vi "CH_LM App DisplayDataFromFile.vi"(0 "Path":path) -> ()   [LabVIEW 2012, in "CH_LM App.lvlib"]
doc: "This VI opens a data file reads the contents and displays them on the frontpanel."
uses:
  CH_LM App.lvlib
  <vilib>/Analysis/NI_AALBase.lvlib
  CH_LM.lvlib
panel:
  out "Table":string[][](table)
  out "Statistics":T1 {"Max" format="%#_4p"; "Min" format="%#_4p"; "Std.Dev." format="%#_4p"; "Mean" format="%#_4p"}
  in  "column":u8
  in  "Statistics Type":T2 {"Max" format="%#_4p"; "Min" format="%#_4p"; "Std. Dev." format="%#_4p"; "Mean" format="%#_4p"}
  out "Statistics Array":T3(array[cluster]) {"Max" format="%#_4p"; "Min" format="%#_4p"; "Std. Dev." format="%#_4p"; "Mean" format="%#_4p"}
  out "Waveform Graph":dbl[][](graph)
  in  "Print":bool
  out "Date and Time":string
  in  "Close":bool
  out "Data file":path
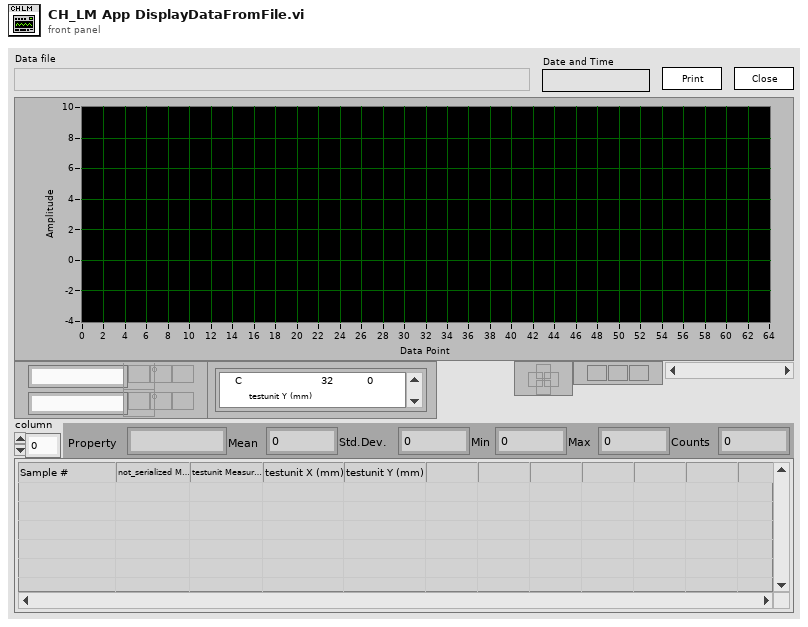
[diagram p1: front panel]
types:
  T1 = cluster{"Property":string, "Mean":dbl, "Std.Dev.":dbl, "Min":dbl, "Max":dbl, "Counts":i32}
  T2 = cluster{"Serial":string, "Mean":dbl, "Std. Dev.":dbl, "Min":dbl, "Max":dbl, "Counts":i32}
  T3 = cluster{"Serial":string, "Mean":dbl, "Std. Dev.":dbl, "Min":dbl, "Max":dbl, "Counts":i32}[]
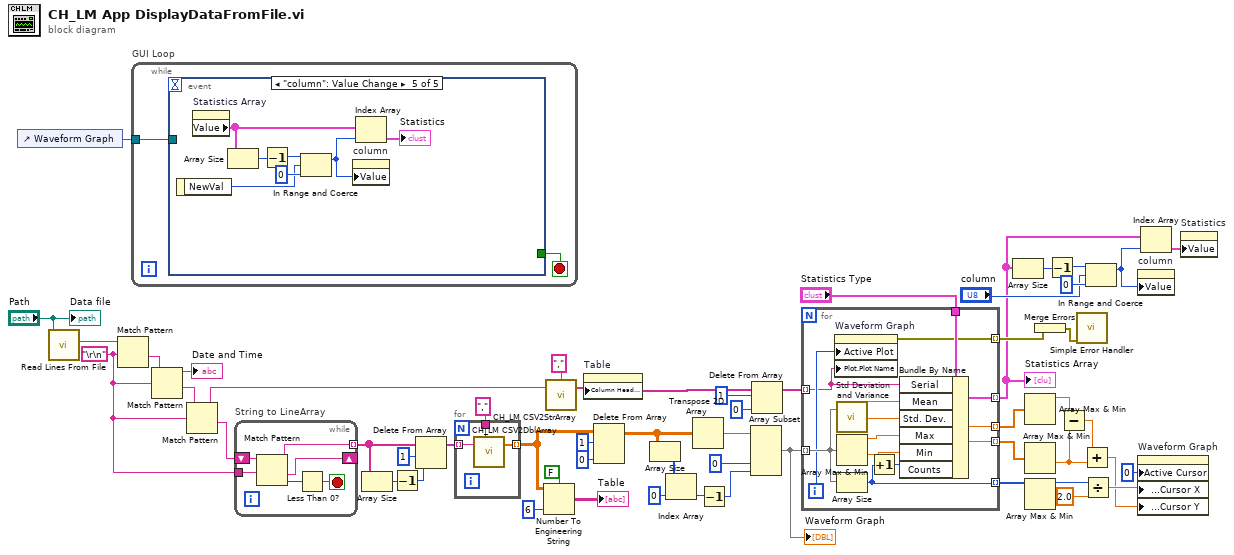
[diagram p0: block diagram]
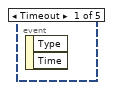
[diagram p2: hidden frame]
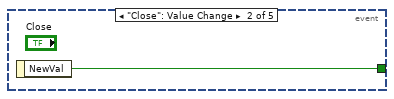
[diagram p3: hidden frame]
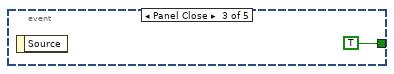
[diagram p4: hidden frame]
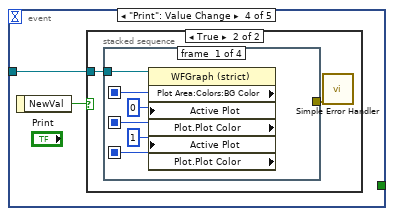
[diagram p5: hidden frame]
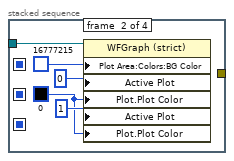
[diagram p7: hidden frame]
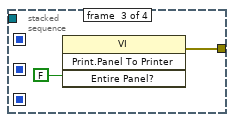
[diagram p8: hidden frame]
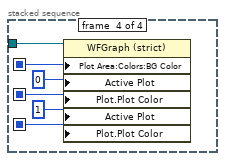
[diagram p9: hidden frame]
diagram:
  w19 = "\r\n" ("End of Line Constant")
  n1 = control-ref of="Waveform Graph"() -> (w50:refnum<vi>)
  n2 = call <vilib>:"Read Lines From File.vi"("file path (dialog if empty)"="Path") -> ("line string"=w54:string)  [unwired: 1 in, 7 out]
  n3 = Match Pattern(string=w54, regular expression=w19) -> (after substring=w53:string)  [unwired: 4 out]
  n4 = while "GUI Loop" {
    tunnel: w50 -> [w56]
    stop <- w57 stop-if-true
    n5 = event shown="[4] \"column\": Value Change" {
      selector: _ -> [_ _ _ _ _]
      dyn-events: _ -> [_ _ _ _ _]
      timeout: _ -> [_ _ _ _ _]
      tunnel: [_ w58 TRUE ("NewVal") _ _] -> w57
      tunnel: w56 -> [_ _ _ w60 _]
      event Timeout {
        n6 = event-data() -> ()  [unwired: 3 out]
      }
      event "Close": Value Change {
        n7 = event-data() -> ("NewVal"=w58:bool)  [unwired: 1 out]
      }
      event Panel Close {
        n8 = event-data() -> ()  [unwired: 2 out]
      }
      event "Print": Value Change {
        n9 = event-data() -> ("NewVal"=w61:bool)  [unwired: 1 out]
        n10 = case shown="True" w61 {
          tunnel: w60 -> [_ w62]
          frame False {
          }
          frame True {
            n11 = stacked-sequence {
              seq-local: [w66 _ _ _] -> [_ _ _ w81]
              seq-local: [w65 _ _ _] -> [_ _ _ w79]
              seq-local: [w64 _ _ _] -> [_ _ _ w77]
              tunnel: [_ _ w75 _] -> w63
              tunnel: w62 -> [w69 w74 _ w82]
              frame #0 {
                n12 = property class="WFGraph (strict)"(reference=w69, "Active Plot"=u32 0, "Active Plot"=u32 1) -> ("Plot Area:Colors:BG Color"=w66:u32, "Plot.Plot Color"=w65:u32, "Plot.Plot Color"=w64:u32)  [unwired: 1 in, 2 out]
              }
              frame #1 {
                w70 = u32 0 ("Plot Area:Colors:BG Color")
                n13 = property class="WFGraph (strict)"(reference=w74, "Plot Area:Colors:BG Color"=u32 16777215, "Active Plot"=u32 0, "Plot.Plot Color"=w70, "Active Plot"=u32 1, "Plot.Plot Color"=w70) -> ()  [unwired: 1 in, 2 out]
              }
              frame #2 {
                n14 = invoke on="Invoke Node" class="VI" method="Print.Panel To Printer"("Entire Panel?"=FALSE) -> (error out=w75:errorcluster)  [unwired: 3 in, 3 out]
              }
              frame #3 {
                n15 = property class="WFGraph (strict)"(reference=w82, "Plot Area:Colors:BG Color"=w81, "Active Plot"=u32 0, "Plot.Plot Color"=w79, "Active Plot"=u32 1, "Plot.Plot Color"=w77) -> ()  [unwired: 1 in, 2 out]
              }
            }
            n16 = call <vilib>:"Simple Error Handler.vi"("error in (no error)"=w63) -> ()  [unwired: 1 in, 8 out]
          }
        }
      }
      event "column": Value Change {
        n17 = event-data() -> ("NewVal"=w83:u8)  [unwired: 1 out]
        n18 = property on="Statistics Array" class="Arr (strict)"() -> ("Value"=w86:T3)  [unwired: 2 in, 2 out]
        n19 = Array Size(array=w86) -> (size(s)=w89:i32)
        n20 = Decrement(x=w89) -> (x-1=w88:i32)
        n21 = In Range and Coerce(upper limit=w88, x=w83, lower limit=0) -> (coerced(x)=w85:i32)  [unwired: 1 out]
        n22 = property on="column" class="DigNum (strict)"("Value"=w85) -> ()  [unwired: 2 in, 2 out]
        n23 = Index Array(array=w86, index=w85) -> (element=→"Statistics":T2)
      }
    }
  }
  n24 = Match Pattern(string=w53, regular expression=w19) -> (before substring=→"Date and Time":string, after substring=w52:string)  [unwired: 3 out]
  n25 = Match Pattern(string=w52, regular expression=w19) -> (before substring=w28:string, after substring=w18:string)  [unwired: 3 out]
  n26 = while "String to LineArray" {
    shift-right: [w93] -> _
    shift-left: w18 -> [w95]
    tunnel: w19 -> [w94]
    tunnel: [w90] -> w3 mode=indexing
    stop <- w91 stop-if-true
    n27 = Match Pattern(string=w95, regular expression=w94) -> (before substring=w90:string, after substring=w93:string, offset past match=w92:i32)  [unwired: 2 out]
    n28 = Less Than 0?(x=w92) -> (x < 0?=w91:bool)
  }
  n29 = Array Size(array=w3) -> (size(s)=w2:i32)
  n30 = Decrement(x=w2) -> (x-1=w1:i32)
  n31 = Delete From Array(array=w3, length=1, index=w1) -> (array with subset deleted=w5:string[])  [unwired: 1 out]
  n32 = for {
    tunnel: w5 -> [w98] mode=indexing
    tunnel: "," ("delimiter (Tab)") -> [w97]
    tunnel: [w96] -> w16 mode=indexing
    n33 = call "CH_LM CSV2DblArray.vi"("CSL"=w98, "Separator (,)"=w97) -> ("Double array"=w96:dbl[])  [unwired: 2 in, 1 out]
  }
  n34 = Number To Engineering String(1:FALSE ("use system decimal point (T)"), 2:i16 6 ("precision (6)"), 4:w16) -> (0:→"Table":string[][])  [unwired: 1 out]
  n35 = call "CH_LM CSV2StrArray.vi"("CSL"=w28, "Separator (,)"="," ("delimiter (Tab)")) -> ("Strings"=w23:string[])  [unwired: 1 in, 1 out]
  n36 = property on="Table" class="Tbl (strict)"("Column Header Strings[]"=w23) -> ()  [unwired: 2 in, 2 out]
  n37 = Delete From Array(array=w16, length=1, index (col)=0 ("disabled index (col)")) -> (array with subset deleted=w26:dbl[][])  [unwired: 1 in, 1 out]
  n38 = Array Size(array=w26) -> (size(s)=w37:i32[])
  n39 = Index Array(array=w37, index=0) -> (element=w35:i32)
  n40 = Transpose 2D Array(2D array=w26) -> (transposed array=w32:dbl[][])
  n41 = Decrement(x=w35) -> (x-1=w33:i32)
  n42 = Array Subset(array=w32, index (col)=0 ("index"), length (col)=w33) -> (w15:dbl[][])  [unwired: 2 in]
  "Waveform Graph" <- w15
  n43 = Delete From Array(array=w23, length=1, index=0) -> (array with subset deleted=w22:string[])  [unwired: 1 out]
  n44 = for {
    tunnel: [w106] -> w45 mode=indexing
    tunnel: w15 -> [w110] mode=indexing
    tunnel: "Statistics Type" -> [w109]
    tunnel: w22 -> [w100] mode=indexing
    tunnel: [w105] -> w7 mode=indexing
    tunnel: [w104] -> w44 mode=indexing
    tunnel: [w103] -> w39 mode=indexing
    tunnel: [w101] -> w14 mode=indexing
    i -> [w102]
    n45 = property on="Waveform Graph" class="WFGraph (strict)"("Active Plot"=w102, "Plot.Plot Name"=w100) -> (error out=w101:errorcluster)  [unwired: 2 in, 1 out]
    n46 = call <vilib>:"Std Deviation and Variance.vi"("X"=w110) -> ("mean"=w108:dbl, "standard deviation"=w107:dbl)  [unwired: 1 in, 1 out]
    n47 = Array Max & Min(array=w110) -> (max value=w104:dbl, min value=w103:dbl)  [unwired: 2 out]
    n48 = Array Size(array=w110) -> (size(s)=w106:i32)
    n49 = Increment(x=w106) -> (x+1=w99:i32)
    n50 = Bundle By Name(cluster=w109, "Serial"=w100, "Mean"=w108, "Std. Dev."=w107, "Max"=w104, "Min"=w103, "Counts"=w99) -> (w105:T2)
  }
  "Statistics Array" <- w7
  n51 = Array Size(array=w7) -> (size(s)=w9:i32)
  n52 = Array Max & Min(array=w44) -> (max value=w40:dbl)  [unwired: 3 out]
  n53 = Array Max & Min(array=w39) -> (min value=w38:dbl)  [unwired: 3 out]
  n54 = Array Max & Min(array=w45) -> (max value=w46:i32)  [unwired: 3 out]
  n55 = Merge Errors(w14) -> (w13:errorcluster)
  n56 = Decrement(x=w9) -> (x-1=w10:i32)
  n57 = Subtract(x=w40, y=w38) -> (x-y=w42:dbl)
  n58 = call <vilib>:"Simple Error Handler.vi"("error in (no error)"=w13) -> ()  [unwired: 1 in, 8 out]
  n59 = Add(x=w42, y=w38) -> (x+y=w41:dbl)
  n60 = Divide(x=w46, y=2.0) -> (x/y=w48:dbl)
  n61 = In Range and Coerce(upper limit=w10, x="column", lower limit=0) -> (coerced(x)=w12:i32)  [unwired: 1 out]
  n62 = property on="column" class="DigNum (strict)"("Value"=w12) -> ()  [unwired: 2 in, 2 out]
  n63 = property on="Waveform Graph" class="WFGraph (strict)"("Active Cursor"=u32 0, "Cursor.Cursor Position:Cursor X"=w48, "Cursor.Cursor Position:Cursor Y"=w41) -> ()  [unwired: 2 in, 2 out]
  n64 = Index Array(array=w7, index=w12) -> (element=w6:T2)
  n65 = property on="Statistics" class="Clust (strict)"("Value"=w6) -> ()  [unwired: 2 in, 2 out]
  "Data file" <- "Path"
